vi "svl_Build x and y Axes.vi"(3 "y0 and delta y":cluster{"y0":dbl, "delta y":dbl} {"delta y" format="%.2f"; "y0" format="%.2f"}, 4 "x0 and delta x":cluster{"x0":dbl, "delta x":dbl} {"delta x" format="%.2f"; "x0" format="%.2f"}, 5 "size(s)":i32[](array[numeric])) -> (0 "y autoscale":cluster{"y min":dbl, "y max":dbl} {"y max" format="%.2f"; "y min" format="%.2f"}, 1 "x autoscale":cluster{"x min":dbl, "x max":dbl} {"x max" format="%.2f"; "x min" format="%.2f"}, 2 "scale info":cluster{"x scale":dbl[], "y scale":dbl[]} {"y scale" format="%.2f"; "x scale" format="%.2f"})   [LabVIEW 2017]
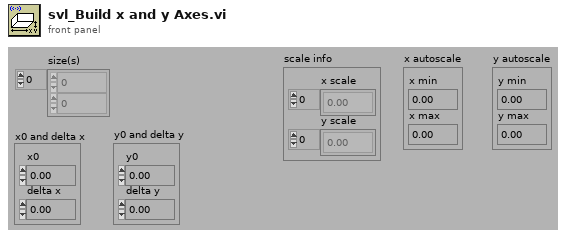
[diagram p1: front panel]
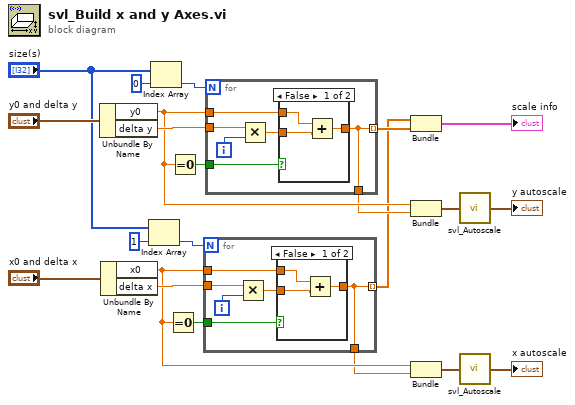
[diagram p0: block diagram]
diagram:
  n1 = Unbundle By Name("y0 and delta y") -> ("y0"=w11:dbl, "delta y"=w17:dbl)
  n2 = Unbundle By Name("x0 and delta x") -> ("x0"=w9:dbl, "delta x"=w18:dbl)
  n3 = Index Array(array="size(s)", index=1) -> (element=w20:i32)
  n4 = Index Array(array="size(s)", index=0) -> (element=w15:i32)
  n5 = Equal To 0?(x=w9) -> (x = 0?=w19:bool)
  n6 = Equal To 0?(x=w11) -> (x = 0?=w16:bool)
  n7 = for {
    N: w20 -> [_]
    tunnel: w19 -> [w28]
    tunnel: w18 -> [w27]
    tunnel: w9 -> [w24]
    tunnel: [w23] -> w5 mode=indexing
    tunnel: [w23] -> w8
    i -> [w26]
    n8 = Multiply(x=w27, y=w26) -> (x*y=w25:dbl)
    n9 = case shown="False" w28 {
      tunnel: w25 -> [w31 w32]
      tunnel: w24 -> [w30 _]
      tunnel: [w29 w32] -> w23
      frame False {
        n10 = Add(x=w30, y=w31) -> (x+y=w29:dbl)
      }
      frame True {
      }
    }
  }
  n11 = for {
    N: w15 -> [_]
    tunnel: w16 -> [w38]
    tunnel: w17 -> [w37]
    tunnel: w11 -> [w34]
    tunnel: [w33] -> w6 mode=indexing
    tunnel: [w33] -> w10
    i -> [w36]
    n12 = Multiply(x=w37, y=w36) -> (x*y=w35:dbl)
    n13 = case shown="False" w38 {
      tunnel: w35 -> [w41 w42]
      tunnel: w34 -> [w40 _]
      tunnel: [w39 w42] -> w33
      frame False {
        n14 = Add(x=w40, y=w41) -> (x+y=w39:dbl)
      }
      frame True {
      }
    }
  }
  n15 = Bundle(w5, w6) -> (→"scale info":cluster{dbl[], dbl[]})  [unwired: 1 in]
  n16 = Bundle("y0"=w11, w10) -> (w4:cluster{"y0":dbl, dbl})  [unwired: 1 in]
  n17 = Bundle("x0"=w9, w8) -> (w3:cluster{"x0":dbl, dbl})  [unwired: 1 in]
  n18 = call <vilib>:"svl_Autoscale.vi"("scale"=w4) -> ("autoscale"=→"y autoscale":cluster{"min":dbl, "max":dbl})
  n19 = call <vilib>:"svl_Autoscale.vi"("scale"=w3) -> ("autoscale"=→"x autoscale":cluster{"min":dbl, "max":dbl})
